vi "Convert Digital Waveform to analog waveforms (SubVI).vi"(8 "error in (no error)":errorcluster, 10 "Digital waveform in":digitalwaveform[](array[waveform]), 11 "Refnum in":refnum<k21>) -> (0 "error out":errorcluster, 2 "Analog waveform array out":waveform(dbl)[](array[waveform]), 3 "Refnum out":refnum<k21>)   [LabVIEW 2015]
doc: "This VI is designed to take a digital waveform from a daq task, determine the number of channels in the task then extract those digital data channels and output an array of analog waveforms that can be plotted on a waveorm graph or chart."
uses:
  <vilib>/Waveform/DWDTOps.llb/DWDT Digital Signal Subset.vi
  <vilib>/Waveform/DWDTOps.llb/DWDT Digital to Analog.vi
  <resource>/objmgr/daqmx.rc
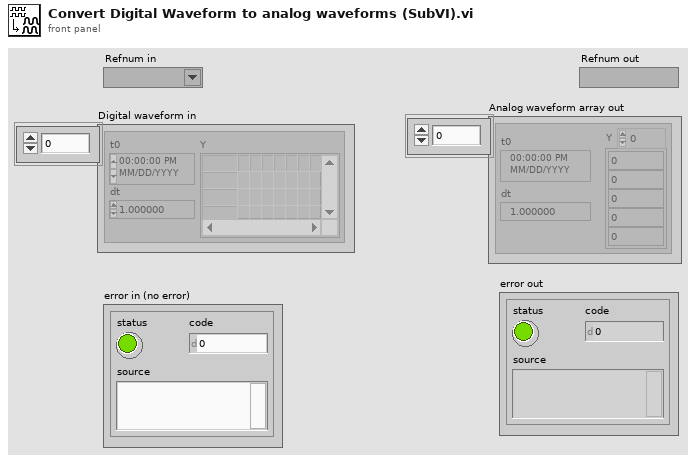
[diagram p1: front panel]
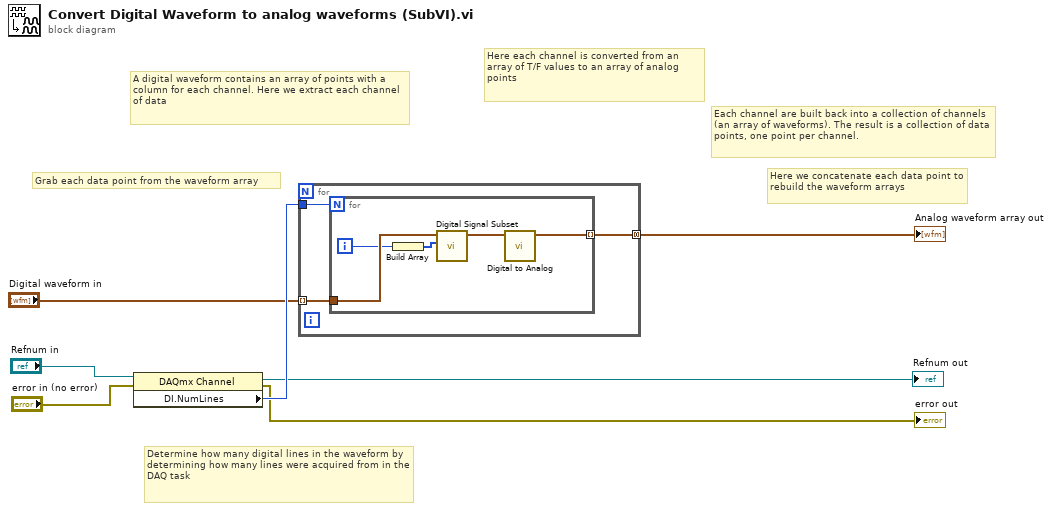
[diagram p0: block diagram]
diagram:
  # "Here we concatenate each data point to rebuild the waveform arrays"
  # "Each channel are built back into a collection of channels (an array of waveforms). The result is a collection of data points, one point per channel."
  # "Here each channel is converted from an array of T/F values to an array of analog points"
  # "A digital waveform contains an array of points with a column for each channel. Here we extract each channel of data"
  # "Grab each data point from the waveform array"
  # "Determine how many digital lines in the waveform by determining how many lines were acquired from in the DAQ task"
  n1 = property class="DAQmx Channel"(reference="Refnum in", error in="error in (no error)") -> (reference out=→"Refnum out":refnum<k21>, error out=→"error out":errorcluster, "DI.NumLines"=w6:u32)
  n2 = for {
    tunnel: "Digital waveform in" -> [w10] mode=indexing
    tunnel: [w9] -> w7 mode=concatenating
    tunnel: w6 -> [w8]
    n3 = for {
      N: w8 -> [_]
      tunnel: w10 -> [w15]
      tunnel: [w12] -> w9 mode=indexing
      i -> [w11]
      n4 = Build Array(w11) -> (w13:i32[])
      n5 = call-poly <vilib>:"Digital Signal Subset.vi"("signals"=w13, "digital waveform"=w15) -> ("digital subset"=w14:digitalwaveform)  [unwired: 8 in, 1 out]
      n6 = call-poly <vilib>:"Digital to Analog.vi"("digital waveform"=w14) -> ("analog waveform"=w12:waveform(dbl))  [unwired: 7 in, 3 out]
    }
  }
  "Analog waveform array out" <- w7
